vi "_Create Event.vi"(9 "Event":refnum<class "Event jettl.lvclass">, 10 "Self Event Alias":string) -> (3 "Create Event Msg Strategy out":refnum<class "Create Event Msg Strategy.lvclass">)   [LabVIEW 2021, in "jettl Msg Create Event.lvlib"]
uses:
  jettl Msg Create Event.lvlib
  Create Event Msg Strategy/Create Event Msg Strategy.lvclass
  jettl/Event jettl/Event jettl.lvclass
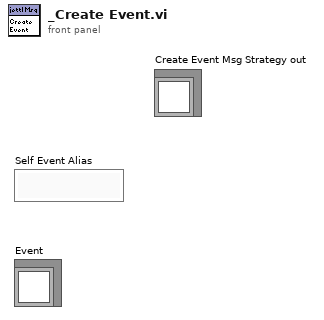
[diagram p1: front panel]
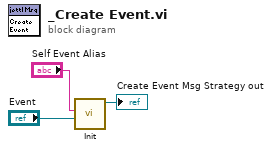
[diagram p0: block diagram]
diagram:
  n1 = call "Init.vi"("Event"="Event", "Self Event Alias"="Self Event Alias") -> ("Create Event Msg Strategy out"=→"Create Event Msg Strategy out":refnum<class "Create Event Msg Strategy.lvclass">)  [unwired: 9 in]
